vi "buildWorkerConfigure.vi"(8 "error in (no error)":errorcluster, 11 "BuildServer in":refnum<class "BuildServer.lvclass">) -> (0 "error out":errorcluster, 3 "BuildServer out":refnum<class "BuildServer.lvclass">)   [LabVIEW 2017, in "BuildServer.lvlib" / "BuildServer.lvclass"]
uses:
  BuildServer.lvclass
  BuildWorker/Classes/BuildWorker/BuildWorker.lvclass
  BuildServer.lvclass/BuildServer.ctl
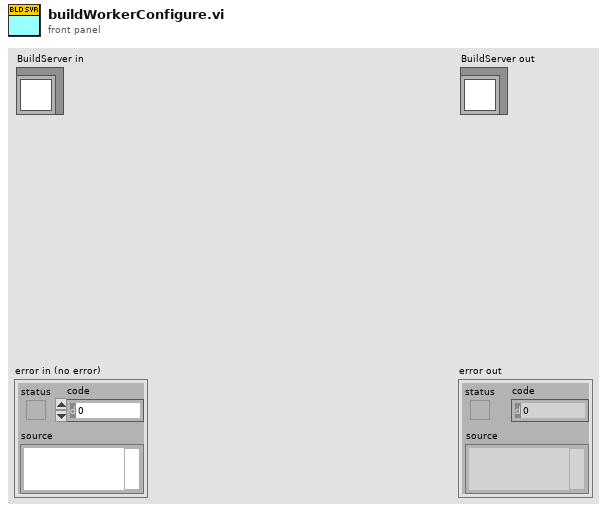
[diagram p1: front panel]
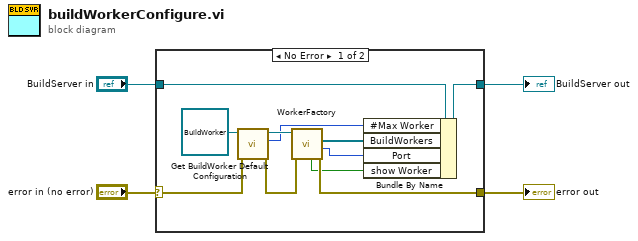
[diagram p0: block diagram]
diagram:
  n1 = case shown="No Error" "error in (no error)" {
    selector: "error in (no error)" -> [w14 w17]
    tunnel: [w7 w17] -> w3
    tunnel: [w13 w16] -> w1
    tunnel: "BuildServer in" -> [w15 w16]
    frame No Error {
      n2 = call-dynamic "Get BuildWorker Default Configuration.vi"("error in (no error)"=w14, "BuildWorker in"=refnum<class "BuildWorker.lvclass"> refnum ("BuildWorker Controller in")) -> ("error out"=w8:errorcluster, "#Max Worker"=w10:i32, "BuildWorker out"=w11:refnum<class "BuildWorker.lvclass">)  [unwired: 7 in]
      n3 = call "WorkerFactory.vi"("error in (no error)"=w8, "BuildWorker in"=w11) -> ("error out"=w7:errorcluster, "Port"=w6:u16, "BuildWorkers"=w9:refnum<class "BuildWorker.lvclass">[], "Show"=w5:bool)  [unwired: 5 in, 1 out]
      n4 = Bundle By Name(cluster=w15, "#Max Worker"=w10, "BuildWorkers"=w9, "Port"=w6, "show Worker"=w5) -> (w13:refnum<class "BuildServer.lvclass">)
    }
    frame Error {
    }
  }
  "error out" <- w3
  "BuildServer out" <- w1
